vi "PID_Globals_Acquires.vi"() -> ()   [LabVIEW 2016]
panel:
  in  "FTot PID gains":cluster{"P":dbl, "I":dbl, "D":dbl}={"P"=1.0, "I"=0.01, "D"=0.0} {"D" format="%.3f"; "I" format="%.3f"; "P" format="%.3f"}
  in  "F1 PID gains":cluster{"P":dbl, "I":dbl, "D":dbl}={"P"=1.0, "I"=0.01, "D"=0.0} {"D" format="%.3f"; "I" format="%.3f"; "P" format="%.3f"}
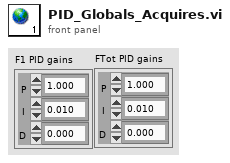
[diagram p1: front panel]
diagram:
